vi "SerialCommunicationTestDevice.vi"() -> ()   [LabVIEW 2020]
doc: "LabVIEW example of communication with simple device which can measure some undefined parameter. Transmitted data in the form of ASCII command. Works with Arduino Uno with SerialCommunicationTestDevice_Arduino code. Comments in Polish."
uses:
  9f4190a0-4c6a-405f-8297-6b348ee77e95.vi
  <vilib>/Instr/_visa.llb/VISA Configure Serial Port (Instr).vi
  <vilib>/Utility/error.llb/Error Cluster From Error Code.vi
  <vilib>/regexp/Match Regular Expression.xnode
  <vilib>/ErrorRing/Error Ring.xnode
panel:
  out "Error out":errorcluster
  in  "stop bits (10: 1 bit)":u16(ring)=10 caption="Liczba bitów stopu" items=["1.0"=10, "1.5"=15, "2.0"=20]
  in  "timeout (10sec)":u32=10000 caption="Timeout"
  in  "parity (0:none)":enum16{"None", "Odd", "Even", "Mark", "Space"}(ring) caption="Bit parzystości"
  in  "data bits (8)":u16=8 caption="Liczba bitów w ramce"
  in  "baud rate (9600)":u32=9600 caption="Szybkość transmisji"
  in  "VISA resource name":refnum<visa-resource-name>="COM7" caption="Port do komunikacji"
  out "Ok close?":bool caption="Urzadzenie poprawnie zamknięte"
  out "Data":string caption="Pomiary z urządzenia"
  in  "Measure":bool
  in  "stop":bool
  out "Ok set?":bool=TRUE caption="Urządzenie gotowe"
  out "DeviceID":string caption="ID urządzenia"
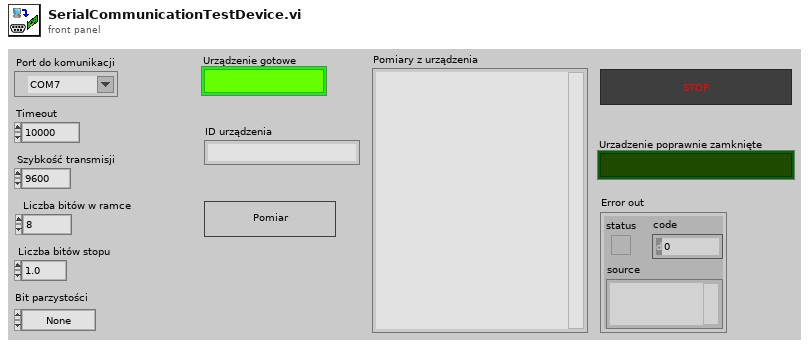
[diagram p1: front panel]
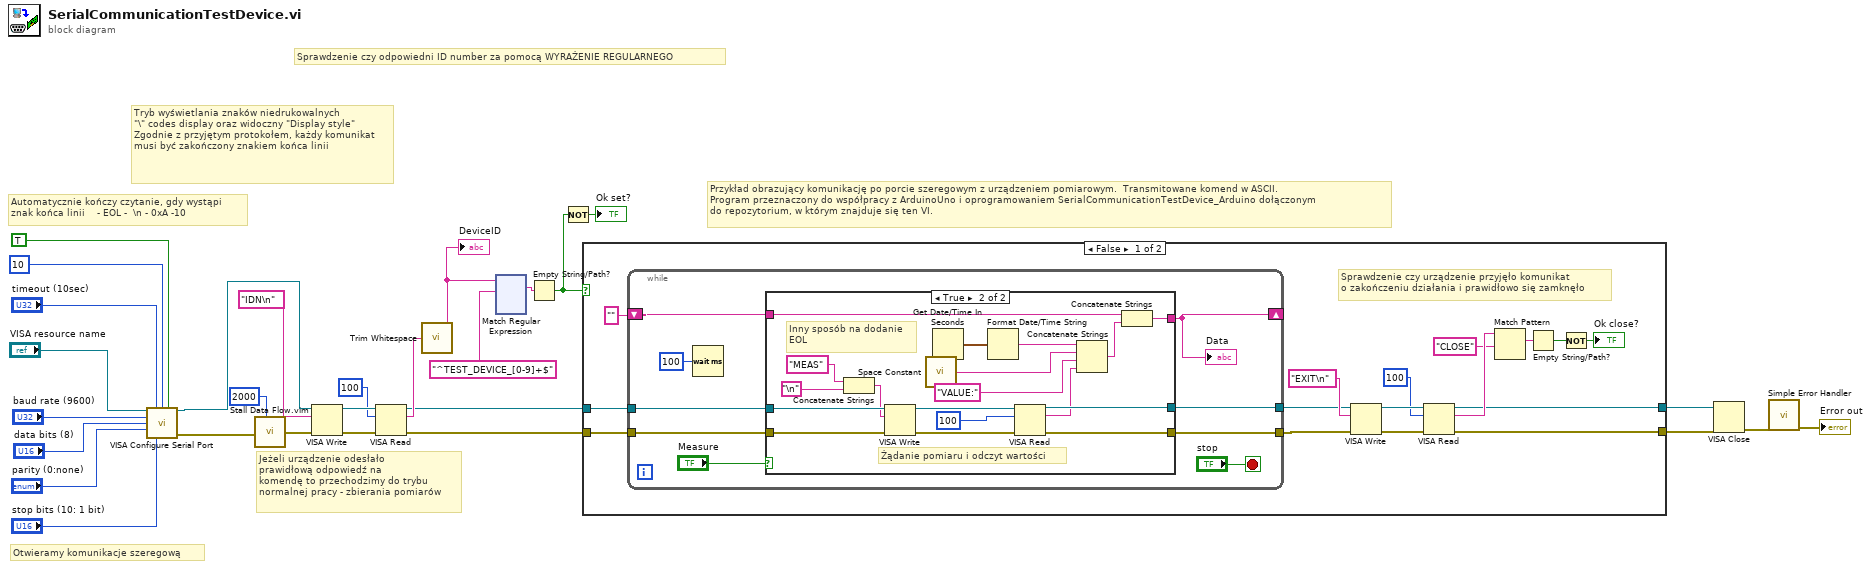
[diagram p0: block diagram]
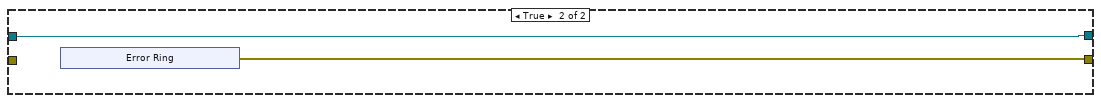
[diagram p3: hidden frame]
diagram:
  # "Przykład obrazujący komunikację po porcie szeregowym z urządzeniem pomiarowym.  Transmitowane komend w ASCII. \nProgram przeznaczony do współpracy z ArduinoUno i oprogramowaniem SerialCommunicationTestDevice_Arduino dołączonym \ndo repozytorium, w którym znajduje się ten VI."
  # "Sprawdzenie czy odpowiedni ID number za pomocą WYRAŻENIE REGULARNEGO"
  # "Jeżeli urządzenie odesłało \nprawidłową odpowiedź na \nkomendę to przechodzimy do trybu\nnormalnej pracy - zbierania pomiarów"
  # "Automatycznie kończy czytanie, gdy wystąpi\nznak końca linii    - EOL -  \\n - 0xA -10"
  # "Tryb wyświetlania znaków niedrukowalnych\n\"\\\" codes display oraz widoczny \"Display style\"\nZgodnie z przyjętym protokołem, każdy komunikat musi być zakończony znakiem końca linii"
  # "Otwieramy komunikacje szeregową"
  n1 = call-poly "VISA Configure Serial Port"("VISA resource name"="VISA resource name", "timeout (10sec)"="timeout (10sec)", "termination char\n(0xA = '\\n' = LF)"=u8 10 ("termination char\n(0xA = '\\n' = LF)"), "Enable Termination\nChar (T)"=TRUE ("Enable Termination\nChar (T)"), "baud rate (9600)"="baud rate (9600)", "data bits (8)"="data bits (8)", "parity (0:none)"="parity (0:none)", "stop bits (10: 1 bit)"="stop bits (10: 1 bit)") -> ("VISA resource name out"=w8:refnum<visa-resource-name>, "error out"=w7:errorcluster)  [unwired: 6 in]
  n2 = call "Stall Data Flow.vim"("value in"=w7, "milliseconds to wait"=u32 2000) -> ("value out"=w28:errorcluster)  [unwired: 1 out]
  n3 = VISA Write(VISA resource name=w8, write buffer="IDN\n", error in (no error)=w28) -> (VISA resource name out=w24:refnum<visa-resource-name>, error out=w25:errorcluster)  [unwired: 1 out]
  n4 = VISA Read(VISA resource name=w24, byte count=u32 100, error in (no error)=w25) -> (VISA resource name out=w16:refnum<visa-resource-name>, read buffer=w22:string, error out=w17:errorcluster)  [unwired: 1 out]
  n5 = call <vilib>:"Trim Whitespace.vi"("string"=w22) -> ("trimmed string"=w1:string)  [unwired: 1 in]
  "DeviceID" <- w1
  n6 = xnode "Match Regular Expression"("input string"=w1, "regular expression"="^TEST_DEVICE_[0-9]+$") -> ("whole match"=w20:string)  [unwired: 4 in, 4 out]
  n7 = Empty String/Path?(string/path=w20) -> (empty?=w19:bool)
  n8 = Not(x=w19) -> (.not. x?=→"Ok set?":bool)
  n9 = case shown="False" w19 {
    tunnel: w17 -> [w44 _]
    tunnel: w16 -> [w43 w76]
    tunnel: [w30 w75] -> w3
    tunnel: [w29 w76] -> w2
    frame False {
      # "Sprawdzenie czy urządzenie przyjęło komunikat\no zakończeniu działania i prawidłowo się zamknęło"
      n10 = while {
        tunnel: w44 -> [w51]
        tunnel: w43 -> [w52]
        tunnel: [w50] -> w33
        tunnel: [w49] -> w31
        shift-right: [w46] -> _
        shift-left: "" -> [w48]
        stop <- "stop" stop-if-true
        n11 = Wait (ms)(milliseconds to wait=u32 100) -> ()  [unwired: 1 out]
        n12 = case shown="True" "Measure" {
          tunnel: w52 -> [w55 w73]
          tunnel: w51 -> [w56 w74]
          tunnel: [w56 w71] -> w50
          tunnel: [w55 w69] -> w49
          tunnel: w48 -> [w54 w61]
          tunnel: [w54 w60] -> w46
          frame False {
            # "Kiedy użytkownik, nie podjemuje akcji o pomiarze\nbrak akcji"
          }
          frame True {
            # "Żądanie pomiaru i odczyt wartości"
            # "Inny sposób na dodanie\nEOL"
            n13 = Concatenate Strings("MEAS" ("string"), "\n") -> (w67:string)
            n14 = VISA Write(VISA resource name=w73, write buffer=w67, error in (no error)=w74) -> (VISA resource name out=w70:refnum<visa-resource-name>, error out=w72:errorcluster)  [unwired: 1 out]
            n15 = call <vilib>:"Space Constant.vi"() -> ("String"=w64:string)
            n16 = Get Date/Time In Seconds() -> (seconds since 1Jan1904=w63:timestamp)
            n17 = Format Date/Time String(seconds (now)=w63) -> (date/time string=w62:string)  [unwired: 2 in]
            n18 = VISA Read(VISA resource name=w70, byte count=u32 100, error in (no error)=w72) -> (VISA resource name out=w69:refnum<visa-resource-name>, read buffer=w68:string, error out=w71:errorcluster)  [unwired: 1 out]
            n19 = Concatenate Strings(w62, w64, "VALUE:" ("string"), w68) -> (w59:string)
            n20 = Concatenate Strings(w61, w59) -> (w60:string)
          }
        }
        "Data" <- w46
      }
      n21 = VISA Write(VISA resource name=w31, write buffer="EXIT\n", error in (no error)=w33) -> (VISA resource name out=w37:refnum<visa-resource-name>, error out=w36:errorcluster)  [unwired: 1 out]
      n22 = VISA Read(VISA resource name=w37, byte count=u32 100, error in (no error)=w36) -> (VISA resource name out=w29:refnum<visa-resource-name>, read buffer=w40:string, error out=w30:errorcluster)  [unwired: 1 out]
      n23 = Match Pattern(string=w40, regular expression="CLOSE") -> (match substring=w38:string)  [unwired: 1 in, 3 out]
      n24 = Empty String/Path?(string/path=w38) -> (empty?=w41:bool)
      n25 = Not(x=w41) -> (.not. x?=→"Ok close?":bool)
    }
    frame True {
      n26 = xnode "Error Ring"() -> ("error out"=w75:errorcluster)
    }
  }
  n27 = VISA Close(VISA resource name=w2, error in (no error)=w3) -> (error out=w15:errorcluster)
  n28 = call <vilib>:"Simple Error Handler.vi"("error in (no error)"=w15) -> ("error out"=→"Error out":errorcluster)  [unwired: 4 in, 4 out]
